vi "Element Events.vi"(8 "error in (no error)":errorcluster, 11 "HistorianCharting in":refnum<class "HistorianCharting.lvclass">) -> (0 "error out":errorcluster, 2 "Element Events":refnum<class "Control Event Registrations.lvclass">, 3 "HistorianCharting out":refnum<class "HistorianCharting.lvclass">)   [LabVIEW 2020, in "VolatusGUIElements.lvlib" / "HistorianCharting.lvclass"]
uses:
  HistorianCharting.lvclass
  VolatusGUI/Control Event Registrations/Control Event Registrations.lvclass
  HistorianCharting.lvclass/HistorianCharting.ctl
  C:/dev/lv20CE/relink/lv-volatus/VolatusGUI/GUI Element/GUI Element.lvclass
  C:/dev/lv20CE/relink/lv-volatus/VolatusGUIElements/HistorianCharting/HistorianCharting.lvclass
  C:/dev/lv20CE/relink/lv-volatus/VolatusGUI/OnValueChangeHandler/OnValueChangeHandler.lvclass
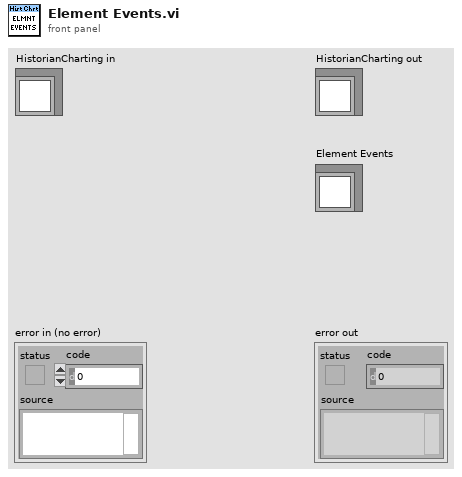
[diagram p1: front panel]
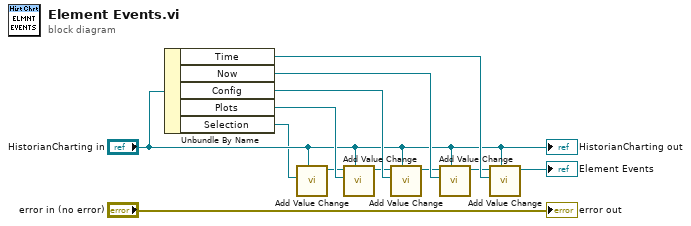
[diagram p0: block diagram]
diagram:
  n1 = Unbundle By Name("HistorianCharting in") -> ("Time"=w10:refnum<vi>, "Now"=w8:refnum<vi>, "Config"=w6:refnum<vi>, "Plots"=w4:refnum<vi>, "Selection"=w1:refnum<vi>)
  n2 = call "Add Value Change.vi"("Control"="HistorianCharting in", "CtlRef"=w1) -> ("Control Event Registrations out"=w3:refnum<class "Control Event Registrations.lvclass">)  [unwired: 8 in, 1 out]
  n3 = call "Add Value Change.vi"("Control"="HistorianCharting in", "CtlRef"=w4, "Control Event Registrations in"=w3) -> ("Control Event Registrations out"=w5:refnum<class "Control Event Registrations.lvclass">)  [unwired: 7 in, 1 out]
  n4 = call "Add Value Change.vi"("Control"="HistorianCharting in", "CtlRef"=w6, "Control Event Registrations in"=w5) -> ("Control Event Registrations out"=w7:refnum<class "Control Event Registrations.lvclass">)  [unwired: 7 in, 1 out]
  n5 = call "Add Value Change.vi"("Control"="HistorianCharting in", "CtlRef"=w8, "Control Event Registrations in"=w7) -> ("Control Event Registrations out"=w9:refnum<class "Control Event Registrations.lvclass">)  [unwired: 7 in, 1 out]
  n6 = call "Add Value Change.vi"("Control"="HistorianCharting in", "CtlRef"=w10, "Control Event Registrations in"=w9) -> ("Control Event Registrations out"=→"Element Events":refnum<class "Control Event Registrations.lvclass">)  [unwired: 7 in, 1 out]
  "error out" <- "error in (no error)"
  "HistorianCharting out" <- "HistorianCharting in"
